vi "(SubVI) Trigger Option for DRC.vi"() -> (1 "DRC trigger option":i32)   [LabVIEW 2014]
panel:
  # "GCS 2.0 must be zero"
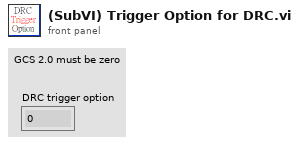
[diagram p1: front panel]
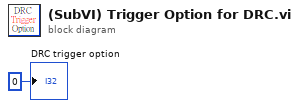
[diagram p0: block diagram]
diagram:
  "DRC trigger option" <- 0
